vi "UV-VIS GetDetector.vi"(0 "UV-VIS in":refnum<class "CCD_camera.lvclass">, 3 "error in (no error)":errorcluster) -> (5 "xpixels":i32, 6 "UV-VIS out":refnum<class "CCD_camera.lvclass">, 7 "ypixels":i32, 8 "DLL error code":u32, 9 "error out":errorcluster)   [LabVIEW 2018, in "CCD_camera.lvclass"]
doc: "This function returns the size of the detector in pixels. The horizontal axis is taken to be the axis parallel to the readout register.\n\n<B>Parameters:</B>\nxpixels - number of horizontal pixels\nypixels - number of vertical pixels\n\n<B>Error codes:</B>\nDRV_SUCCESS - Detector size returned.\nDRV_NOT_INITIALIZED - System not initialized.\nDRV_ACQUIRING - Acquisition in progress."
uses:
  CCD_camera.lvclass
  C:/Users/Sergey Denisov/Documents/REPS/TRANCON/Classes/Detector/Detector.lvclass
  Detector.lvclass/Detector.ctl
  Detector.lvclass
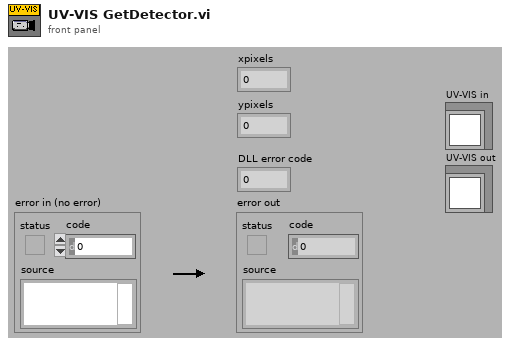
[diagram p1: front panel]
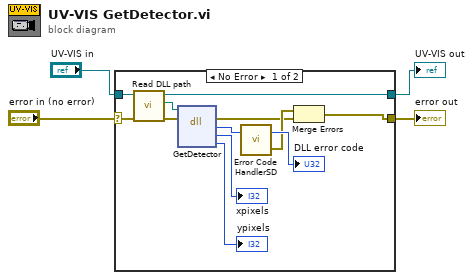
[diagram p0: block diagram]
diagram:
  n1 = case shown="No Error" "error in (no error)" {
    selector: "error in (no error)" -> [w11 w18]
    tunnel: [w6 w18] -> w3
    tunnel: [w5 w17] -> w2
    tunnel: "UV-VIS in" -> [w12 w17]
    frame No Error {
      n2 = call "Read DLL path.vi"("error in (no error)"=w11, "Detector in"=w12) -> ("error out"=w10:errorcluster, "DLL path"=w9:path, "Detector out"=w5:refnum<class "CCD_camera.lvclass">)  [unwired: 7 in]
      n3 = dll-call lib="S:/TRANCON/DLL/Atmcd32d.dll" fn="GetDetector"(path in=w9, error in=w10) -> (error out=w7:errorcluster, "return type"=w16:u32, "xpixels"=→"xpixels":i32, "ypixels"=→"ypixels":i32)  [unwired: 3 in, 1 out]
      n4 = call "Error Code HandlerSD.vi"("DLL error code"=w16) -> ("error out"=w8:errorcluster, "dup DLL error code"=→"DLL error code":u32)  [unwired: 1 in]
      n5 = Merge Errors(w8, w7) -> (w6:errorcluster)
    }
    frame Error {
    }
  }
  "error out" <- w3
  "UV-VIS out" <- w2
